vi "Find New Tunnel.vi"(8 "error in (no error)":errorcluster, 10 "new tunnels in":refnum<vi>[](array[refnum]), 11 "old tunnels in":refnum<vi>[](array[refnum])) -> (0 "error out":errorcluster, 2 "new tunnel":refnum<vi>, 3 "old tunnels out":refnum<vi>[](array[refnum]))   [LabVIEW 2017]
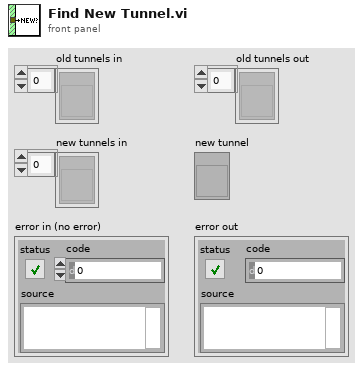
[diagram p1: front panel]
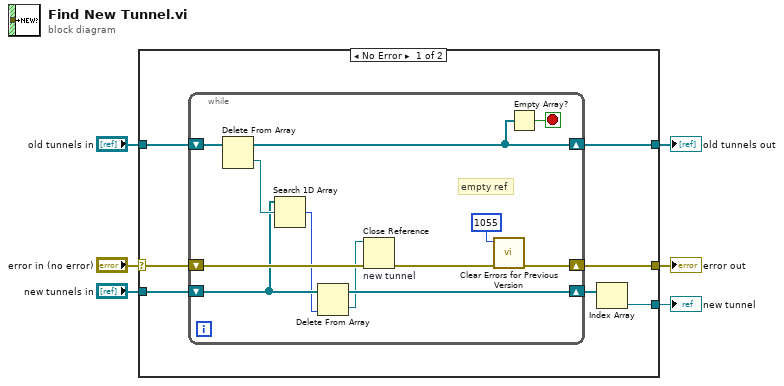
[diagram p0: block diagram]
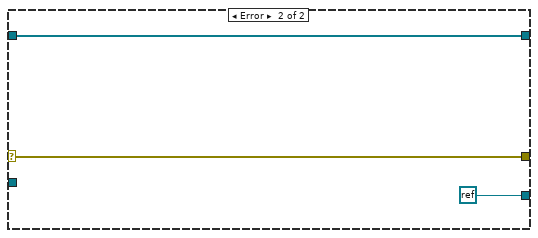
[diagram p2: hidden frame]
diagram:
  n1 = case shown="No Error" "error in (no error)" {
    selector: "error in (no error)" -> [w7 w27]
    tunnel: [w13 refnum<k0> refnum] -> w6
    tunnel: "old tunnels in" -> [w12 w28]
    tunnel: "new tunnels in" -> [w11 _]
    tunnel: [w9 w27] -> w3
    tunnel: [w8 w28] -> w2
    frame No Error {
      n2 = while {
        shift-right: [w23] -> w8
        shift-left: w12 -> [w24]
        shift-right: [w18] -> w10
        shift-left: w11 -> [w20]
        shift-right: [w14] -> w9
        shift-left: w7 -> [w25]
        stop <- w22 stop-if-true
        # "empty ref"
        n3 = Delete From Array(array=w24) -> (deleted portion=w21:refnum<vi>, array with subset deleted=w23:refnum<vi>[])  [unwired: 2 in]
        n4 = Search 1D Array(1D array=w20, element=w21) -> (index of element=w19:i32)  [unwired: 1 in]
        n5 = Delete From Array(array=w20, index=w19) -> (deleted portion=w17:refnum<vi>, array with subset deleted=w18:refnum<vi>[])  [unwired: 1 in]
        n6 = Close Reference "new tunnel"(reference=w17, error in (no error)=w25) -> (error out=w15:errorcluster)
        n7 = call "Clear Errors for Previous Version.vi"("error in (no error)"=w15, "code"=1055) -> ("error out"=w14:errorcluster)  [unwired: 9 in]
        n8 = Empty Array?(array=w23) -> (empty?=w22:bool)
      }
      n9 = Index Array(array=w10) -> (element=w13:refnum<vi>)  [unwired: 1 in]
    }
    frame Error {
    }
  }
  "new tunnel" <- w6
  "error out" <- w3
  "old tunnels out" <- w2
